vi "BRig_RT__Case_Exp__State_initTrial__LC_Cue__v4.vi"(6 "input_arrTrig":bool[](array[boolean]), 8 "input_dataTrial":u16[][](array[numeric]), 9 "input_dataExp":u16[](array[numeric]), 10 "input_dataLC":u16[](array[numeric]), 11 "input_dataCurrent":u16[](array[numeric])) -> (0 "output_dataTrial":u16[][](array[numeric]), 3 "output_dataCurrent":u16[](array[numeric]), 4 "output_arrTrig":bool[](array[boolean]))   [LabVIEW 2014]
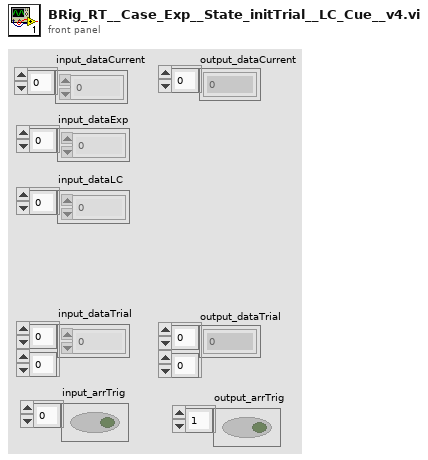
[diagram p1: front panel]
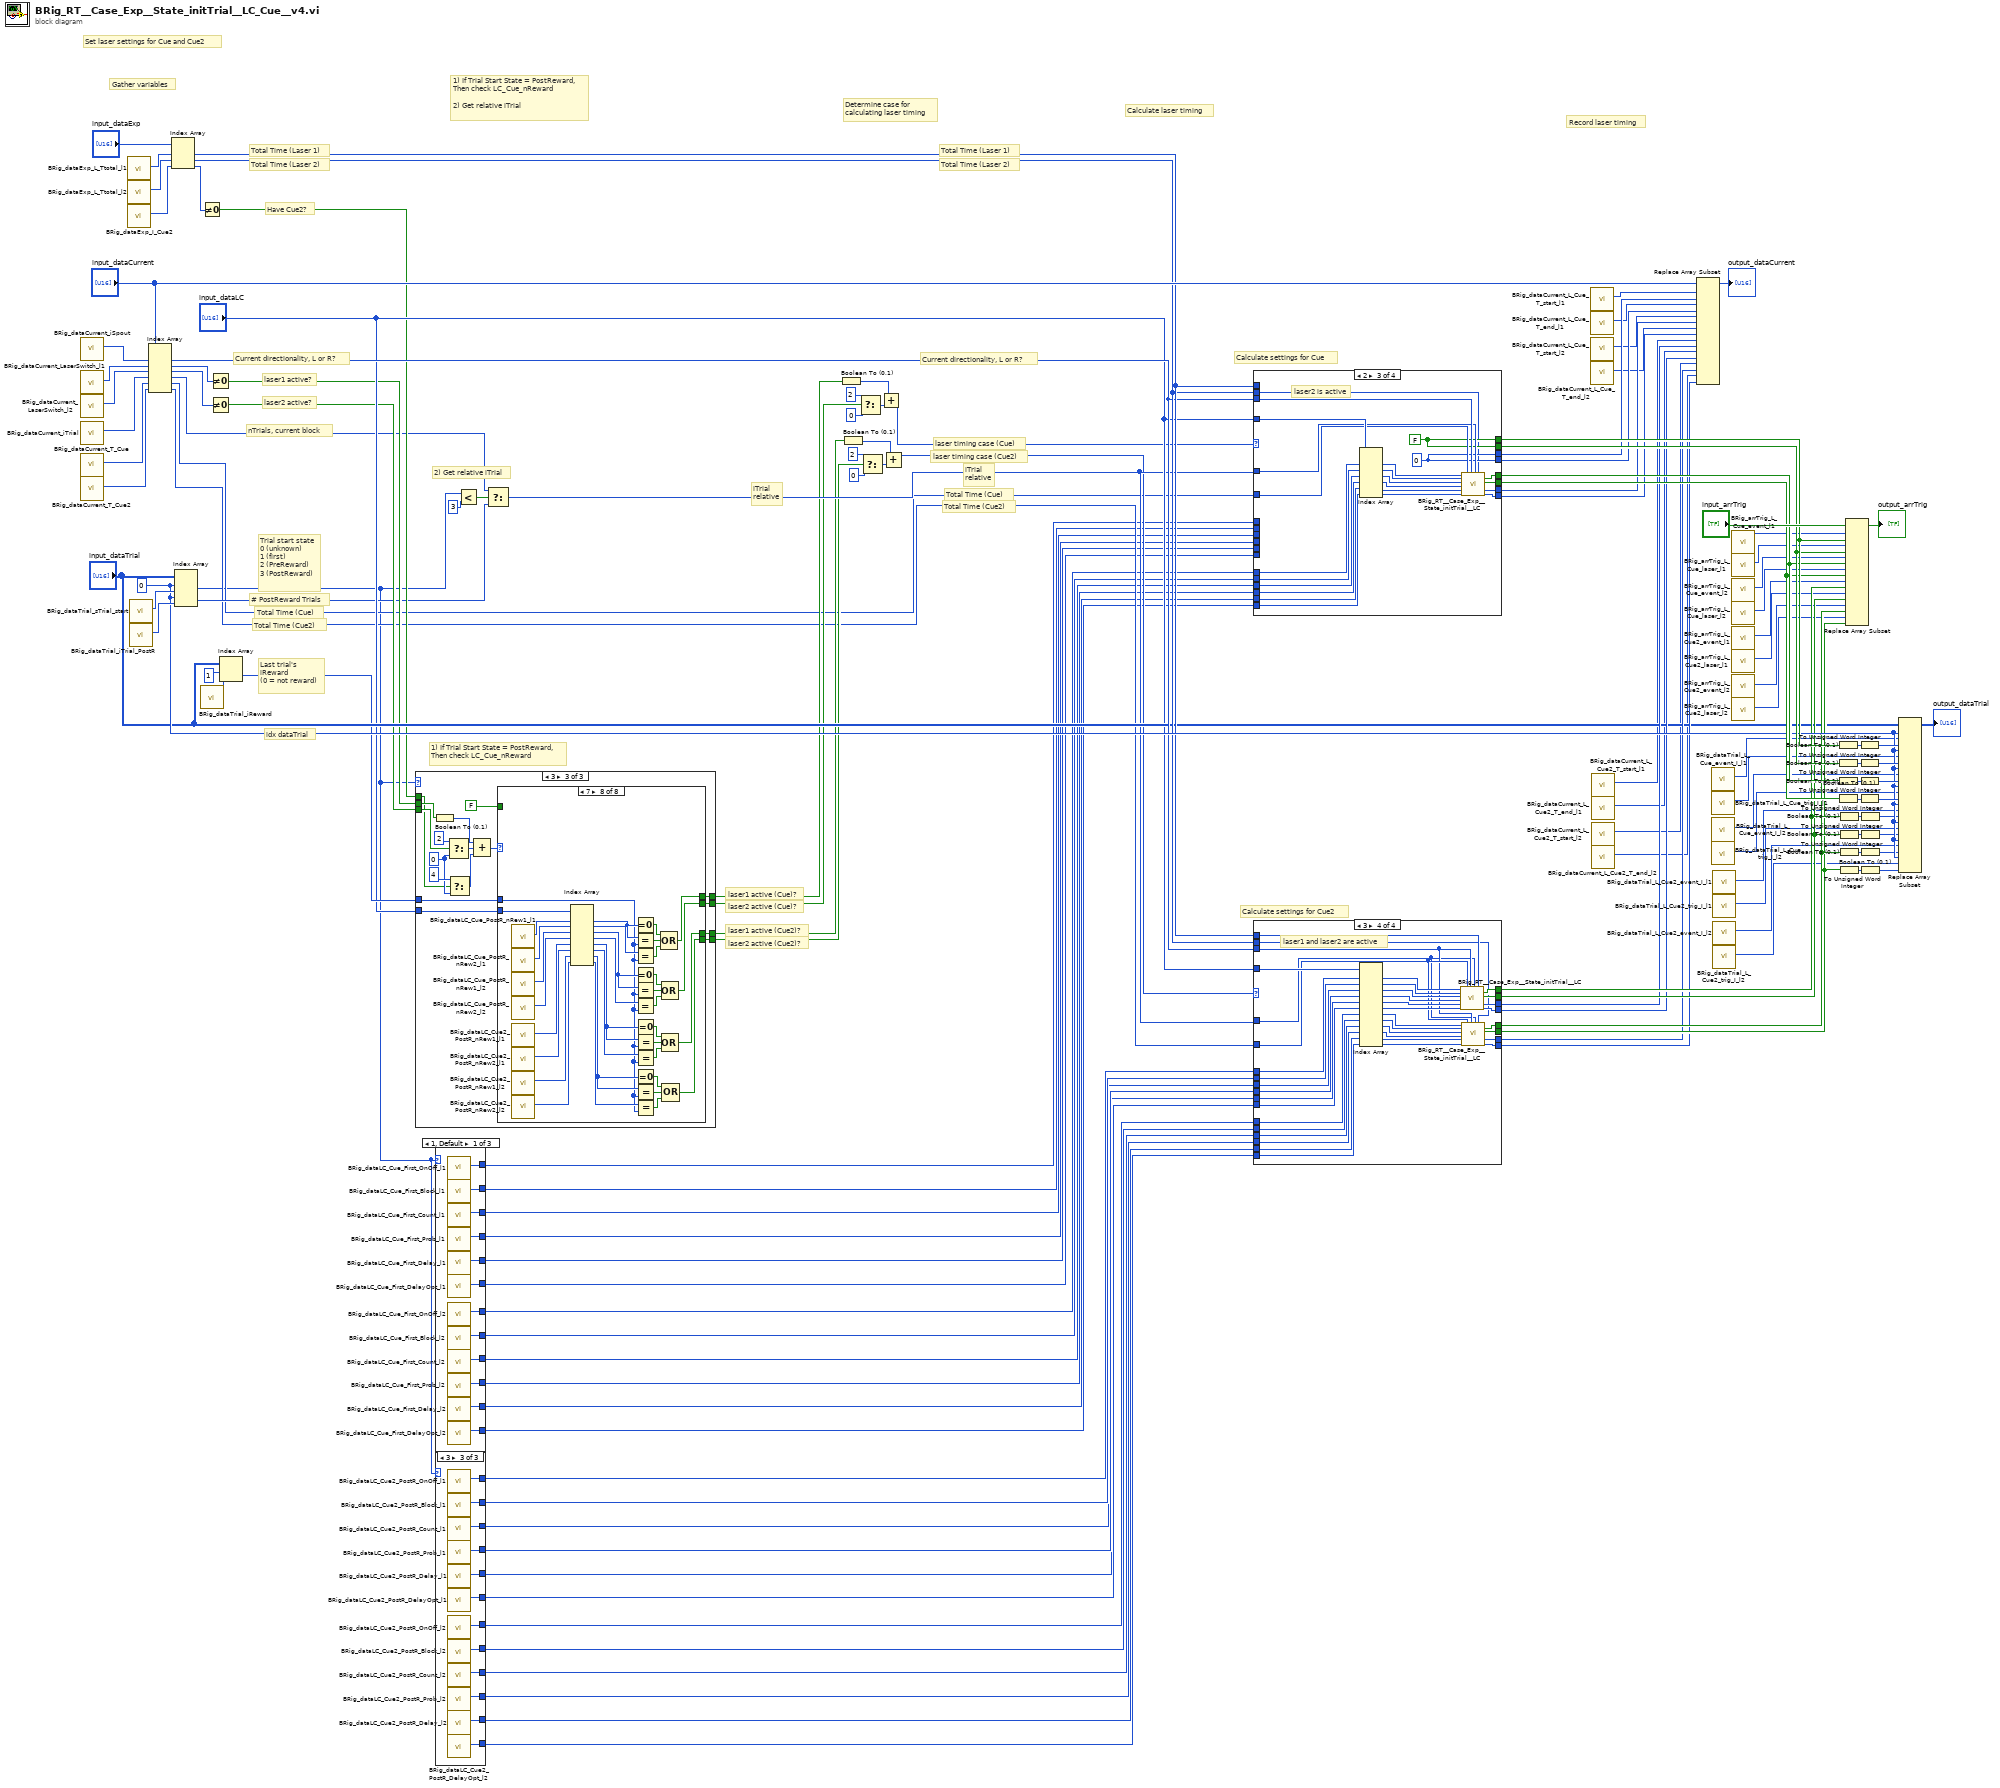
[diagram p0: block diagram]
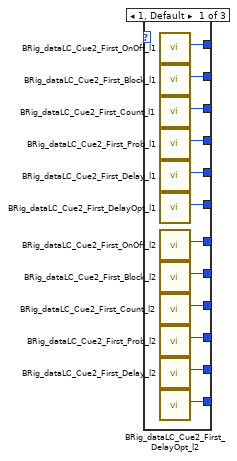
[diagram p2: hidden frame]
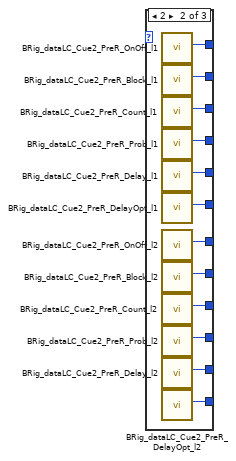
[diagram p3: hidden frame]
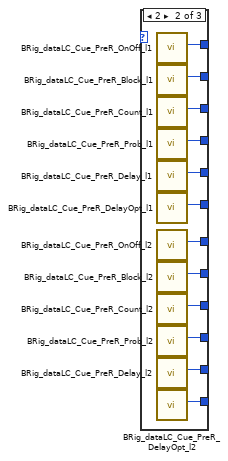
[diagram p4: hidden frame]
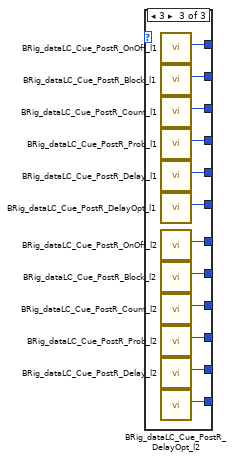
[diagram p5: hidden frame]
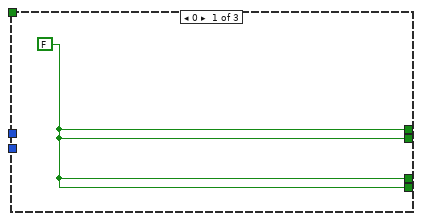
[diagram p6: hidden frame]
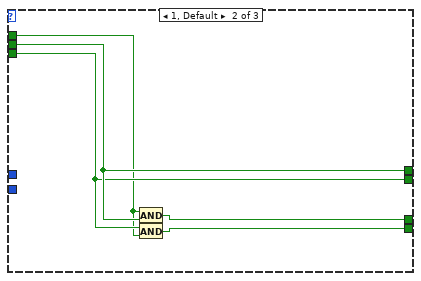
[diagram p7: hidden frame]
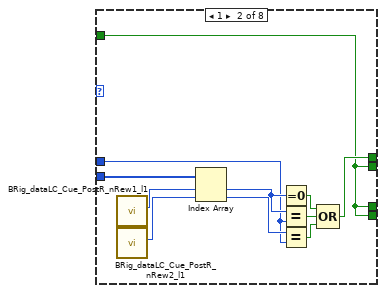
[diagram p9: hidden frame]
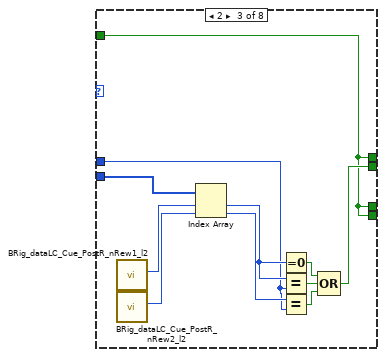
[diagram p10: hidden frame]
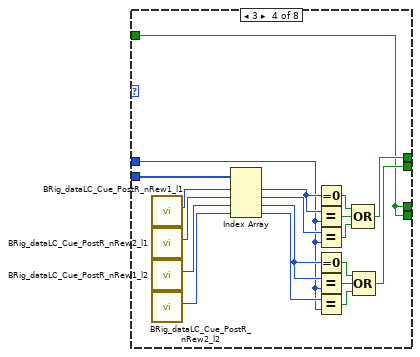
[diagram p11: hidden frame]
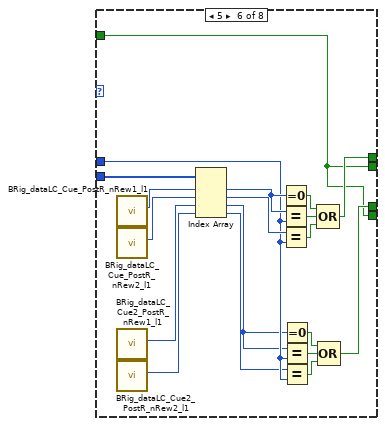
[diagram p13: hidden frame]
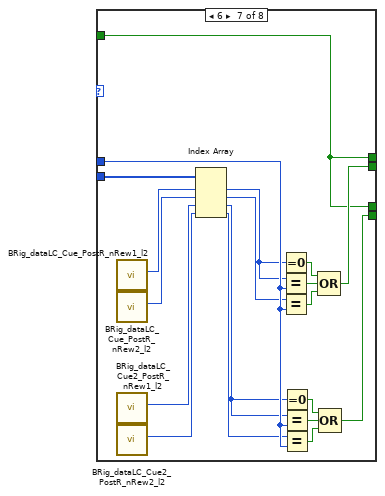
[diagram p14: hidden frame]
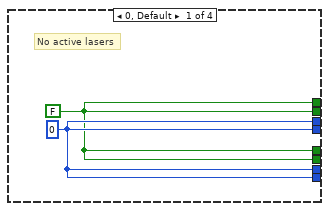
[diagram p15: hidden frame]
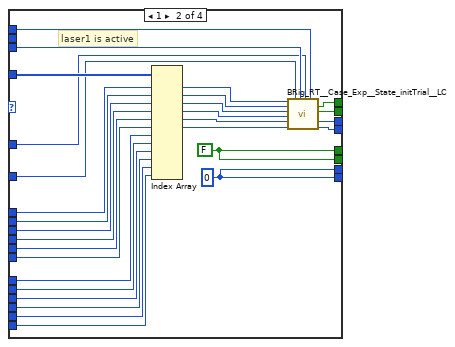
[diagram p16: hidden frame]
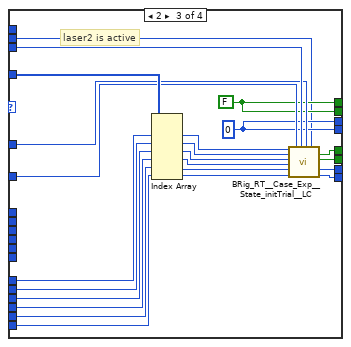
[diagram p17: hidden frame]
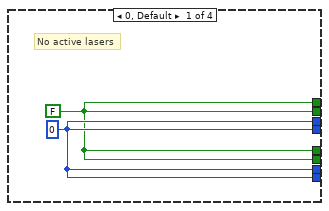
[diagram p18: hidden frame]
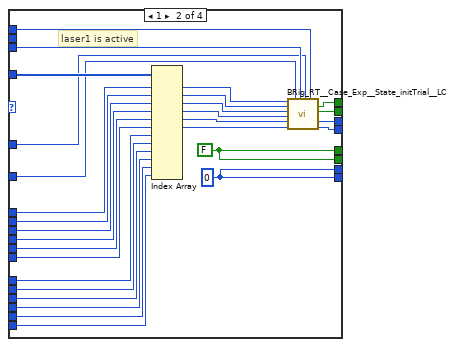
[diagram p19: hidden frame]
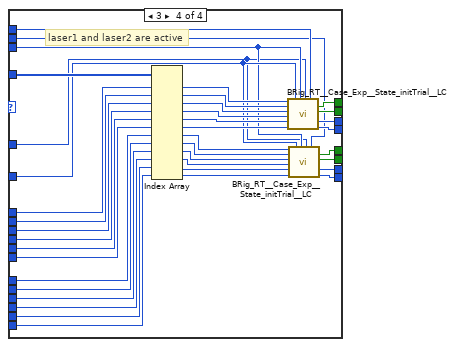
[diagram p20: hidden frame]
diagram:
  w94 = 0
  # "Record laser timing"
  # "Calculate laser timing"
  # "Total Time (Cue2)"
  # "Total Time (Cue)"
  # "iTrial\nrelative"
  # "Total Time (Laser 2)"
  # "Total Time (Laser 1)"
  # "Current directionality, L or R?"
  # "laser timing case (Cue2)"
  # "Determine case for\ncalculating laser timing"
  # "2) Get relative iTrial"
  # "1) If Trial Start State = PostReward,\nThen check LC_Cue_nReward"
  # "laser2 active (Cue2)?"
  # "laser1 active (Cue2)?"
  # "laser2 active (Cue)?"
  # "laser1 active (Cue)?"
  # "1) If Trial Start State = PostReward,\nThen check LC_Cue_nReward\n\n2) Get relative iTrial"
  # "Gather variables"
  # "Last trial's\niReward\n(0 = not reward)"
  # "nTrials, current block"
  # "idx dataTrial"
  # "Total Time (Cue2)"
  # "Total Time (Cue)"
  # "# PostReward Trials"
  # "Current directionality, L or R?"
  # "Have Cue2?"
  # "Total Time (Laser 2)"
  # "Total Time (Laser 1)"
  # "Calculate settings for Cue2"
  # "Calculate settings for Cue"
  # "Set laser settings for Cue and Cue2"
  # "iTrial\nrelative"
  # "laser timing case (Cue)"
  # "Trial start state\n0 (unknown)\n1 (first)\n2 (PreReward)\n3 (PostReward)"
  # "laser2 active?"
  # "laser1 active?"
  n1 = call "BRig_dataCurrent_iSpout.vi"() -> ("output_iSpout"=w125:i32)  [unwired: 11 in]
  n2 = call "BRig_dataCurrent_LaserSwitch_l1.vi"() -> ("output_LaserSwitch_l1"=w134:i32)  [unwired: 11 in]
  n3 = call "BRig_dataCurrent_LaserSwitch_l2.vi"() -> ("output_LaserSwitch_l2"=w133:i32)  [unwired: 11 in]
  n4 = call "BRig_dataCurrent_iTrial.vi"() -> ("output_iTrial"=w99:i32)  [unwired: 11 in]
  n5 = call "BRig_dataCurrent_T_Cue.vi"() -> ("output_T_Cue"=w53:i32)  [unwired: 11 in]
  n6 = call "BRig_dataCurrent_T_Cue2.vi"() -> ("output_T_Cue2"=w52:i32)  [unwired: 11 in]
  n7 = call "BRig_dataExp_L_Ttotal_l1.vi"() -> ("output_L_Ttotal_l1"=w102:i32)  [unwired: 11 in]
  n8 = call "BRig_dataExp_L_Ttotal_l2.vi"() -> ("output_L_Ttotal_l2"=w103:i32)  [unwired: 11 in]
  n9 = call "BRig_dataExp_I_Cue2.vi"() -> ("output_I_Cue2"=w78:i32)  [unwired: 11 in]
  n10 = call "BRig_dataTrial_sTrial_start.vi"() -> ("output_sTrial_start"=w130:i32)  [unwired: 11 in]
  n11 = call "BRig_dataTrial_iTrial_PostR.vi"() -> ("output_iTrial_PostR"=w100:i32)  [unwired: 11 in]
  n12 = Index Array(array="input_dataCurrent", index #1=w125, index #2=w134, index #3=w133, index #4=w99, index #5=w53, index #6=w52) -> (element #1=w87:u16, element #2=w132:u16, element #3=w131:u16, element #4=w66:u16, element #5=w51:u16, element #6=w50:u16)
  n13 = Index Array(array="input_dataExp", index #1=w102, index #2=w103, index #3=w78) -> (element #1=w89:u16, element #2=w88:u16, element #3=w77:u16)
  n14 = Index Array(array="input_dataTrial", index (row) #1=w94, index (col) #1=w130, index (row) #2=w94, index (col) #2=w100) -> (element #1=w25:u16, element #2=w65:u16)
  n15 = Not Equal To 0?(x=w77) -> (x != 0?=w69:bool)
  n16 = call "BRig_dataTrial_iReward.vi"() -> ("output_iReward"=w75:i32)  [unwired: 11 in]
  n17 = Not Equal To 0?(x=w132) -> (x != 0?=w70:bool)
  n18 = Not Equal To 0?(x=w131) -> (x != 0?=w71:bool)
  n19 = Index Array(array="input_dataTrial", index (row)=1 ("disabled index (row)"), index (col)=w75) -> (element=w73:u16)
  n20 = case shown="3" w25 {
    tunnel: w73 -> [_ _ w149]
    tunnel: "input_dataLC" -> [_ _ w150]
    tunnel: w71 -> [_ w139 w142]
    tunnel: w70 -> [_ w140 w143]
    tunnel: w69 -> [_ w138 w141]
    tunnel: [w135 w140 w148] -> w63
    tunnel: [w135 w139 w147] -> w62
    tunnel: [w135 w137 w146] -> w57
    tunnel: [w135 w136 w145] -> w56
    frame 0 {
      w135 = FALSE
    }
    frame 1, Default {
      n21 = And(x=w138, y=w140) -> (x .and. y?=w137:bool)
      n22 = And(x=w139, y=w138) -> (x .and. y?=w136:bool)
    }
    frame 3 {
      w155 = i16 0 ("f")
      n23 = Boolean To (0,1)(Boolean=w143) -> (0, 1=w153:i16)
      n24 = Select(t=i16 2, s=w142, f=w155) -> (s? t:f=w154:i16)
      n25 = Select(t=i16 4, s=w141, f=w155) -> (s? t:f=w152:i16)
      n26 = Compound Arithmetic op=ADD(w153, w154, w152) -> (w151:i16)
      n27 = case shown="7" w151 {
        tunnel: w150 -> [_ w164 w175 w189 _ w214 w235 w262]
        tunnel: w149 -> [_ w163 w174 w188 _ w210 w231 w251]
        tunnel: [w158 w162 w172 w187 w200 w209 w228 w250] -> w148
        tunnel: [w158 w161 w173 w186 w200 w207 w230 w249] -> w147
        tunnel: [w158 w161 w172 w185 w200 w208 w228 w248] -> w146
        tunnel: [w158 w161 w172 w185 w200 w207 w229 w247] -> w145
        tunnel: FALSE -> [w158 w161 w172 w185 w200 w207 w228 _]
        frame 0, Default {
        }
        frame 1 {
          n28 = call "BRig_dataLC_Cue_PostR_nRew1_l1.vi"() -> ("output_Cue_PostR_nRew1_l1"=w159:i32)  [unwired: 11 in]
          n29 = call "BRig_dataLC_Cue_PostR_nRew2_l1.vi"() -> ("output_Cue_PostR_nRew2_l1"=w160:i32)  [unwired: 11 in]
          n30 = Index Array(array=w164, index #1=w159, index #2=w160) -> (element #1=w166:u16, element #2=w165:u16)
          n31 = Equal To 0?(x=w166) -> (x = 0?=w167:bool)
          n32 = Equal?(x=w166, y=w163) -> (x = y?=w168:bool)
          n33 = Equal?(x=w165, y=w163) -> (x = y?=w169:bool)
          n34 = Compound Arithmetic op=OR(w167, w168, w169) -> (w162:bool)
        }
        frame 2 {
          n35 = call "BRig_dataLC_Cue_PostR_nRew1_l2.vi"() -> ("output_Cue_PostR_nRew1_l2"=w170:i32)  [unwired: 11 in]
          n36 = call "BRig_dataLC_Cue_PostR_nRew2_l2.vi"() -> ("output_Cue_PostR_nRew2_l2"=w171:i32)  [unwired: 11 in]
          n37 = Index Array(array=w175, index #1=w170, index #2=w171) -> (element #1=w176:u16, element #2=w177:u16)
          n38 = Equal To 0?(x=w176) -> (x = 0?=w179:bool)
          n39 = Equal?(x=w176, y=w174) -> (x = y?=w178:bool)
          n40 = Equal?(x=w177, y=w174) -> (x = y?=w180:bool)
          n41 = Compound Arithmetic op=OR(w179, w178, w180) -> (w173:bool)
        }
        frame 3 {
          n42 = call "BRig_dataLC_Cue_PostR_nRew1_l1.vi"() -> ("output_Cue_PostR_nRew1_l1"=w181:i32)  [unwired: 11 in]
          n43 = call "BRig_dataLC_Cue_PostR_nRew2_l1.vi"() -> ("output_Cue_PostR_nRew2_l1"=w182:i32)  [unwired: 11 in]
          n44 = call "BRig_dataLC_Cue_PostR_nRew1_l2.vi"() -> ("output_Cue_PostR_nRew1_l2"=w183:i32)  [unwired: 11 in]
          n45 = call "BRig_dataLC_Cue_PostR_nRew2_l2.vi"() -> ("output_Cue_PostR_nRew2_l2"=w184:i32)  [unwired: 11 in]
          n46 = Index Array(array=w189, index #1=w181, index #2=w182, index #3=w183, index #4=w184) -> (element #1=w193:u16, element #2=w192:u16, element #3=w190:u16, element #4=w191:u16)
          n47 = Equal To 0?(x=w193) -> (x = 0?=w194:bool)
          n48 = Equal?(x=w193, y=w188) -> (x = y?=w195:bool)
          n49 = Equal?(x=w192, y=w188) -> (x = y?=w196:bool)
          n50 = Equal To 0?(x=w190) -> (x = 0?=w198:bool)
          n51 = Equal?(x=w190, y=w188) -> (x = y?=w197:bool)
          n52 = Equal?(x=w191, y=w188) -> (x = y?=w199:bool)
          n53 = Compound Arithmetic op=OR(w194, w195, w196) -> (w187:bool)
          n54 = Compound Arithmetic op=OR(w198, w197, w199) -> (w186:bool)
        }
        frame 4 {
        }
        frame 5 {
          n55 = call "BRig_dataLC_Cue_PostR_nRew1_l1.vi"() -> ("output_Cue_PostR_nRew1_l1"=w203:i32)  [unwired: 11 in]
          n56 = call "BRig_dataLC_Cue_PostR_nRew2_l1.vi"() -> ("output_Cue_PostR_nRew2_l1"=w204:i32)  [unwired: 11 in]
          n57 = call "BRig_dataLC_Cue2_PostR_nRew1_l1.vi"() -> ("output_Cue2_PostR_nRew1_l1"=w201:i32)  [unwired: 11 in]
          n58 = call "BRig_dataLC_Cue2_PostR_nRew2_l1.vi"() -> ("output_Cue2_PostR_nRew2_l1"=w202:i32)  [unwired: 11 in]
          n59 = Index Array(array=w214, index #1=w203, index #2=w204, index #3=w201, index #4=w202) -> (element #1=w216:u16, element #2=w215:u16, element #3=w206:u16, element #4=w205:u16)
          n60 = Equal To 0?(x=w216) -> (x = 0?=w217:bool)
          n61 = Equal?(x=w216, y=w210) -> (x = y?=w218:bool)
          n62 = Equal?(x=w215, y=w210) -> (x = y?=w219:bool)
          n63 = Equal To 0?(x=w206) -> (x = 0?=w213:bool)
          n64 = Equal?(x=w206, y=w210) -> (x = y?=w212:bool)
          n65 = Equal?(x=w205, y=w210) -> (x = y?=w211:bool)
          n66 = Compound Arithmetic op=OR(w217, w218, w219) -> (w209:bool)
          n67 = Compound Arithmetic op=OR(w213, w212, w211) -> (w208:bool)
        }
        frame 6 {
          n68 = call "BRig_dataLC_Cue_PostR_nRew1_l2.vi"() -> ("output_Cue_PostR_nRew1_l2"=w223:i32)  [unwired: 11 in]
          n69 = call "BRig_dataLC_Cue_PostR_nRew2_l2.vi"() -> ("output_Cue_PostR_nRew2_l2"=w222:i32)  [unwired: 11 in]
          n70 = call "BRig_dataLC_Cue2_PostR_nRew1_l2.vi"() -> ("output_Cue2_PostR_nRew1_l2"=w221:i32)  [unwired: 11 in]
          n71 = call "BRig_dataLC_Cue2_PostR_nRew2_l2.vi"() -> ("output_Cue2_PostR_nRew2_l2"=w220:i32)  [unwired: 11 in]
          n72 = Index Array(array=w235, index #1=w223, index #2=w222, index #3=w221, index #4=w220) -> (element #1=w227:u16, element #2=w226:u16, element #3=w225:u16, element #4=w224:u16)
          n73 = Equal To 0?(x=w227) -> (x = 0?=w237:bool)
          n74 = Equal?(x=w227, y=w231) -> (x = y?=w236:bool)
          n75 = Equal?(x=w226, y=w231) -> (x = y?=w238:bool)
          n76 = Equal To 0?(x=w225) -> (x = 0?=w233:bool)
          n77 = Equal?(x=w225, y=w231) -> (x = y?=w234:bool)
          n78 = Equal?(x=w224, y=w231) -> (x = y?=w232:bool)
          n79 = Compound Arithmetic op=OR(w237, w236, w238) -> (w230:bool)
          n80 = Compound Arithmetic op=OR(w233, w234, w232) -> (w229:bool)
        }
        frame 7 {
          n81 = call "BRig_dataLC_Cue_PostR_nRew1_l1.vi"() -> ("output_Cue_PostR_nRew1_l1"=w243:i32)  [unwired: 11 in]
          n82 = call "BRig_dataLC_Cue_PostR_nRew2_l1.vi"() -> ("output_Cue_PostR_nRew2_l1"=w244:i32)  [unwired: 11 in]
          n83 = call "BRig_dataLC_Cue_PostR_nRew1_l2.vi"() -> ("output_Cue_PostR_nRew1_l2"=w245:i32)  [unwired: 11 in]
          n84 = call "BRig_dataLC_Cue_PostR_nRew2_l2.vi"() -> ("output_Cue_PostR_nRew2_l2"=w246:i32)  [unwired: 11 in]
          n85 = call "BRig_dataLC_Cue2_PostR_nRew1_l1.vi"() -> ("output_Cue2_PostR_nRew1_l1"=w242:i32)  [unwired: 11 in]
          n86 = call "BRig_dataLC_Cue2_PostR_nRew2_l1.vi"() -> ("output_Cue2_PostR_nRew2_l1"=w241:i32)  [unwired: 11 in]
          n87 = call "BRig_dataLC_Cue2_PostR_nRew1_l2.vi"() -> ("output_Cue2_PostR_nRew1_l2"=w240:i32)  [unwired: 11 in]
          n88 = call "BRig_dataLC_Cue2_PostR_nRew2_l2.vi"() -> ("output_Cue2_PostR_nRew2_l2"=w239:i32)  [unwired: 11 in]
          n89 = Index Array(array=w262, index #1=w243, index #2=w244, index #3=w245, index #4=w246, index #5=w242, index #6=w241, index #7=w240, index #8=w239) -> (element #1=w266:u16, element #2=w265:u16, element #3=w263:u16, element #4=w264:u16, element #5=w255:u16, element #6=w254:u16, element #7=w252:u16, element #8=w253:u16)
          n90 = Equal To 0?(x=w266) -> (x = 0?=w267:bool)
          n91 = Equal?(x=w266, y=w251) -> (x = y?=w268:bool)
          n92 = Equal?(x=w265, y=w251) -> (x = y?=w269:bool)
          n93 = Equal To 0?(x=w263) -> (x = 0?=w271:bool)
          n94 = Equal?(x=w263, y=w251) -> (x = y?=w270:bool)
          n95 = Equal?(x=w264, y=w251) -> (x = y?=w272:bool)
          n96 = Equal To 0?(x=w255) -> (x = 0?=w261:bool)
          n97 = Equal?(x=w255, y=w251) -> (x = y?=w260:bool)
          n98 = Equal?(x=w254, y=w251) -> (x = y?=w259:bool)
          n99 = Equal To 0?(x=w252) -> (x = 0?=w257:bool)
          n100 = Equal?(x=w252, y=w251) -> (x = y?=w258:bool)
          n101 = Equal?(x=w253, y=w251) -> (x = y?=w256:bool)
          n102 = Compound Arithmetic op=OR(w267, w268, w269) -> (w250:bool)
          n103 = Compound Arithmetic op=OR(w271, w270, w272) -> (w249:bool)
          n104 = Compound Arithmetic op=OR(w261, w260, w259) -> (w248:bool)
          n105 = Compound Arithmetic op=OR(w257, w258, w256) -> (w247:bool)
        }
      }
    }
  }
  n106 = case shown="1, Default" w25 {
    tunnel: [w273 w296 w307] -> w38
    tunnel: [w274 w285 w306] -> w39
    tunnel: [w275 w286 w305] -> w40
    tunnel: [w276 w287 w304] -> w41
    tunnel: [w277 w288 w303] -> w42
    tunnel: [w278 w289 w302] -> w43
    tunnel: [w279 w295 w301] -> w44
    tunnel: [w280 w290 w300] -> w45
    tunnel: [w281 w291 w299] -> w46
    tunnel: [w282 w292 w298] -> w47
    tunnel: [w283 w293 w297] -> w48
    tunnel: [w284 w294 w308] -> w49
    frame 1, Default {
      n107 = call "BRig_dataLC_Cue_First_OnOff_l1.vi"() -> ("output_Cue_First_OnOff"=w273:i32)  [unwired: 11 in]
      n108 = call "BRig_dataLC_Cue_First_Block_l1.vi"() -> ("output_Cue_First_Block"=w274:i32)  [unwired: 11 in]
      n109 = call "BRig_dataLC_Cue_First_Count_l1.vi"() -> ("output_Cue_First_Count"=w275:i32)  [unwired: 11 in]
      n110 = call "BRig_dataLC_Cue_First_Prob_l1.vi"() -> ("output_Cue_First_Prob"=w276:i32)  [unwired: 11 in]
      n111 = call "BRig_dataLC_Cue_First_Delay_l1.vi"() -> ("output_Cue_First_Delay"=w277:i32)  [unwired: 11 in]
      n112 = call "BRig_dataLC_Cue_First_DelayOpt_l1.vi"() -> ("output_Cue_First_DelayOpt"=w278:i32)  [unwired: 11 in]
      n113 = call "BRig_dataLC_Cue_First_OnOff_l2.vi"() -> ("output_Cue_First_OnOff_l2"=w279:i32)  [unwired: 11 in]
      n114 = call "BRig_dataLC_Cue_First_Block_l2.vi"() -> ("output_Cue_First_Block_l2"=w280:i32)  [unwired: 11 in]
      n115 = call "BRig_dataLC_Cue_First_Count_l2.vi"() -> ("output_Cue_First_Count_l2"=w281:i32)  [unwired: 11 in]
      n116 = call "BRig_dataLC_Cue_First_Prob_l2.vi"() -> ("output_Cue_First_Prob_l2"=w282:i32)  [unwired: 11 in]
      n117 = call "BRig_dataLC_Cue_First_Delay_l2.vi"() -> ("output_Cue_First_Delay_l2"=w283:i32)  [unwired: 11 in]
      n118 = call "BRig_dataLC_Cue_First_DelayOpt_l2.vi"() -> ("output_Cue_First_DelayOpt_l2"=w284:i32)  [unwired: 11 in]
    }
    frame 2 {
      n119 = call "BRig_dataLC_Cue_PreR_OnOff_l1.vi"() -> ("output_Cue_PreR_OnOff"=w296:i32)  [unwired: 11 in]
      n120 = call "BRig_dataLC_Cue_PreR_Block_l1.vi"() -> ("output_Cue_PreR_Block"=w285:i32)  [unwired: 11 in]
      n121 = call "BRig_dataLC_Cue_PreR_Count_l1.vi"() -> ("output_Cue_PreR_Count"=w286:i32)  [unwired: 11 in]
      n122 = call "BRig_dataLC_Cue_PreR_Prob_l1.vi"() -> ("output_Cue_PreR_Prob"=w287:i32)  [unwired: 11 in]
      n123 = call "BRig_dataLC_Cue_PreR_Delay_l1.vi"() -> ("output_Cue_PreR_Delay"=w288:i32)  [unwired: 11 in]
      n124 = call "BRig_dataLC_Cue_PreR_DelayOpt_l1.vi"() -> ("output_Cue_PreR_DelayOpt"=w289:i32)  [unwired: 11 in]
      n125 = call "BRig_dataLC_Cue_PreR_OnOff_l2.vi"() -> ("output_Cue_PreR_OnOff_l2"=w295:i32)  [unwired: 11 in]
      n126 = call "BRig_dataLC_Cue_PreR_Block_l2.vi"() -> ("output_Cue_PreR_Block_l2"=w290:i32)  [unwired: 11 in]
      n127 = call "BRig_dataLC_Cue_PreR_Count_l2.vi"() -> ("output_Cue_PreR_Count_l2"=w291:i32)  [unwired: 11 in]
      n128 = call "BRig_dataLC_Cue_PreR_Prob_l2.vi"() -> ("output_Cue_PreR_Prob_l2"=w292:i32)  [unwired: 11 in]
      n129 = call "BRig_dataLC_Cue_PreR_Delay_l2.vi"() -> ("output_Cue_PreR_Delay_l2"=w293:i32)  [unwired: 11 in]
      n130 = call "BRig_dataLC_Cue_PreR_DelayOpt_l2.vi"() -> ("output_Cue_PreR_DelayOpt_l2"=w294:i32)  [unwired: 11 in]
    }
    frame 3 {
      n131 = call "BRig_dataLC_Cue_PostR_OnOff_l1.vi"() -> ("output_Cue_PostR_OnOff"=w307:i32)  [unwired: 11 in]
      n132 = call "BRig_dataLC_Cue_PostR_Block_l1.vi"() -> ("output_Cue_PostR_Block"=w306:i32)  [unwired: 11 in]
      n133 = call "BRig_dataLC_Cue_PostR_Count_l1.vi"() -> ("output_Cue_PostR_Count"=w305:i32)  [unwired: 11 in]
      n134 = call "BRig_dataLC_Cue_PostR_Prob_l1.vi"() -> ("output_Cue_PostR_Prob"=w304:i32)  [unwired: 11 in]
      n135 = call "BRig_dataLC_Cue_PostR_Delay_l1.vi"() -> ("output_Cue_PostR_Delay"=w303:i32)  [unwired: 11 in]
      n136 = call "BRig_dataLC_Cue_PostR_DelayOpt_l1.vi"() -> ("output_Cue_PostR_DelayOpt"=w302:i32)  [unwired: 11 in]
      n137 = call "BRig_dataLC_Cue_PostR_OnOff_l2.vi"() -> ("output_Cue_PostR_OnOff_l2"=w301:i32)  [unwired: 11 in]
      n138 = call "BRig_dataLC_Cue_PostR_Block_l2.vi"() -> ("output_Cue_PostR_Block_l2"=w300:i32)  [unwired: 11 in]
      n139 = call "BRig_dataLC_Cue_PostR_Count_l2.vi"() -> ("output_Cue_PostR_Count_l2"=w299:i32)  [unwired: 11 in]
      n140 = call "BRig_dataLC_Cue_PostR_Prob_l2.vi"() -> ("output_Cue_PostR_Prob_l2"=w298:i32)  [unwired: 11 in]
      n141 = call "BRig_dataLC_Cue_PostR_Delay_l2.vi"() -> ("output_Cue_PostR_Delay_l2"=w297:i32)  [unwired: 11 in]
      n142 = call "BRig_dataLC_Cue_PostR_DelayOpt_l2.vi"() -> ("output_Cue_PostR_DelayOpt_l2"=w308:i32)  [unwired: 11 in]
    }
  }
  n143 = case shown="3" w25 {
    tunnel: [w320 w332 w344] -> w37
    tunnel: [w319 w331 w343] -> w36
    tunnel: [w318 w330 w342] -> w35
    tunnel: [w317 w329 w341] -> w34
    tunnel: [w316 w328 w340] -> w33
    tunnel: [w315 w327 w339] -> w32
    tunnel: [w314 w326 w338] -> w31
    tunnel: [w313 w325 w337] -> w30
    tunnel: [w312 w324 w336] -> w29
    tunnel: [w311 w323 w335] -> w28
    tunnel: [w310 w322 w334] -> w27
    tunnel: [w309 w321 w333] -> w26
    frame 1, Default {
      n144 = call "BRig_dataLC_Cue2_First_OnOff_l1.vi"() -> ("output_Cue2_First_OnOff"=w320:i32)  [unwired: 11 in]
      n145 = call "BRig_dataLC_Cue2_First_Block_l1.vi"() -> ("output_Cue2_First_Block"=w319:i32)  [unwired: 11 in]
      n146 = call "BRig_dataLC_Cue2_First_Count_l1.vi"() -> ("output_Cue2_First_Count"=w318:i32)  [unwired: 11 in]
      n147 = call "BRig_dataLC_Cue2_First_Prob_l1.vi"() -> ("output_Cue2_First_Prob"=w317:i32)  [unwired: 11 in]
      n148 = call "BRig_dataLC_Cue2_First_Delay_l1.vi"() -> ("output_Cue2_First_Delay"=w316:i32)  [unwired: 11 in]
      n149 = call "BRig_dataLC_Cue2_First_DelayOpt_l1.vi"() -> ("output_Cue2_First_DelayOpt"=w315:i32)  [unwired: 11 in]
      n150 = call "BRig_dataLC_Cue2_First_OnOff_l2.vi"() -> ("output_Cue2_First_OnOff_l2"=w314:i32)  [unwired: 11 in]
      n151 = call "BRig_dataLC_Cue2_First_Block_l2.vi"() -> ("output_Cue2_First_Block_l2"=w313:i32)  [unwired: 11 in]
      n152 = call "BRig_dataLC_Cue2_First_Count_l2.vi"() -> ("output_Cue2_First_Count_l2"=w312:i32)  [unwired: 11 in]
      n153 = call "BRig_dataLC_Cue2_First_Prob_l2.vi"() -> ("output_Cue2_First_Prob_l2"=w311:i32)  [unwired: 11 in]
      n154 = call "BRig_dataLC_Cue2_First_Delay_l2.vi"() -> ("output_Cue2_First_Delay_l2"=w310:i32)  [unwired: 11 in]
      n155 = call "BRig_dataLC_Cue2_First_DelayOpt_l2.vi"() -> ("output_Cue2_First_DelayOpt_l2"=w309:i32)  [unwired: 11 in]
    }
    frame 2 {
      n156 = call "BRig_dataLC_Cue2_PreR_OnOff_l1.vi"() -> ("output_Cue2_PreR_OnOff"=w332:i32)  [unwired: 11 in]
      n157 = call "BRig_dataLC_Cue2_PreR_Block_l1.vi"() -> ("output_Cue2_PreR_Block"=w331:i32)  [unwired: 11 in]
      n158 = call "BRig_dataLC_Cue2_PreR_Count_l1.vi"() -> ("output_Cue2_PreR_Count"=w330:i32)  [unwired: 11 in]
      n159 = call "BRig_dataLC_Cue2_PreR_Prob_l1.vi"() -> ("output_Cue2_PreR_Prob"=w329:i32)  [unwired: 11 in]
      n160 = call "BRig_dataLC_Cue2_PreR_Delay_l1.vi"() -> ("output_Cue2_PreR_Delay"=w328:i32)  [unwired: 11 in]
      n161 = call "BRig_dataLC_Cue2_PreR_DelayOpt_l1.vi"() -> ("output_Cue2_PreR_DelayOpt"=w327:i32)  [unwired: 11 in]
      n162 = call "BRig_dataLC_Cue2_PreR_OnOff_l2.vi"() -> ("output_Cue2_PreR_OnOff_l2"=w326:i32)  [unwired: 11 in]
      n163 = call "BRig_dataLC_Cue2_PreR_Block_l2.vi"() -> ("output_Cue2_PreR_Block_l2"=w325:i32)  [unwired: 11 in]
      n164 = call "BRig_dataLC_Cue2_PreR_Count_l2.vi"() -> ("output_Cue2_PreR_Count_l2"=w324:i32)  [unwired: 11 in]
      n165 = call "BRig_dataLC_Cue2_PreR_Prob_l2.vi"() -> ("output_Cue2_PreR_Prob_l2"=w323:i32)  [unwired: 11 in]
      n166 = call "BRig_dataLC_Cue2_PreR_Delay_l2.vi"() -> ("output_Cue2_PreR_Delay_l2"=w322:i32)  [unwired: 11 in]
      n167 = call "BRig_dataLC_Cue2_PreR_DelayOpt_l2.vi"() -> ("output_Cue2_PreR_DelayOpt_l2"=w321:i32)  [unwired: 11 in]
    }
    frame 3 {
      n168 = call "BRig_dataLC_Cue2_PostR_OnOff_l1.vi"() -> ("output_Cue2_PostR_OnOff"=w344:i32)  [unwired: 11 in]
      n169 = call "BRig_dataLC_Cue2_PostR_Block_l1.vi"() -> ("output_Cue2_PostR_Block"=w343:i32)  [unwired: 11 in]
      n170 = call "BRig_dataLC_Cue2_PostR_Count_l1.vi"() -> ("output_Cue2_PostR_Count"=w342:i32)  [unwired: 11 in]
      n171 = call "BRig_dataLC_Cue2_PostR_Prob_l1.vi"() -> ("output_Cue2_PostR_Prob"=w341:i32)  [unwired: 11 in]
      n172 = call "BRig_dataLC_Cue2_PostR_Delay_l1.vi"() -> ("output_Cue2_PostR_Delay"=w340:i32)  [unwired: 11 in]
      n173 = call "BRig_dataLC_Cue2_PostR_DelayOpt_l1.vi"() -> ("output_Cue2_PostR_DelayOpt"=w339:i32)  [unwired: 11 in]
      n174 = call "BRig_dataLC_Cue2_PostR_OnOff_l2.vi"() -> ("output_Cue2_PostR_OnOff_l2"=w338:i32)  [unwired: 11 in]
      n175 = call "BRig_dataLC_Cue2_PostR_Block_l2.vi"() -> ("output_Cue2_PostR_Block_l2"=w337:i32)  [unwired: 11 in]
      n176 = call "BRig_dataLC_Cue2_PostR_Count_l2.vi"() -> ("output_Cue2_PostR_Count_l2"=w336:i32)  [unwired: 11 in]
      n177 = call "BRig_dataLC_Cue2_PostR_Prob_l2.vi"() -> ("output_Cue2_PostR_Prob_l2"=w335:i32)  [unwired: 11 in]
      n178 = call "BRig_dataLC_Cue2_PostR_Delay_l2.vi"() -> ("output_Cue2_PostR_Delay_l2"=w334:i32)  [unwired: 11 in]
      n179 = call "BRig_dataLC_Cue2_PostR_DelayOpt_l2.vi"() -> ("output_Cue2_PostR_DelayOpt_l2"=w333:i32)  [unwired: 11 in]
    }
  }
  n180 = Less?(x=w25, y=u16 3) -> (x < y?=w67:bool)
  n181 = Select(t=w66, s=w67, f=w65) -> (s? t:f=w64:u16)
  n182 = Boolean To (0,1)(Boolean=w63) -> (0, 1=w127:i16)
  n183 = Boolean To (0,1)(Boolean=w57) -> (0, 1=w60:i16)
  n184 = Select(t=i16 2, s=w62, f=i16 0) -> (s? t:f=w128:i16)
  n185 = Select(t=i16 2, s=w56, f=i16 0) -> (s? t:f=w59:i16)
  n186 = Add(x=w127, y=w128) -> (x+y=w55:i16)
  n187 = Add(x=w60, y=w59) -> (x+y=w54:i16)
  n188 = case shown="2" w55 {
    tunnel: "input_dataLC" -> [_ w375 w398 w436]
    tunnel: w87 -> [_ w367 w390 w422]
    tunnel: w51 -> [_ w368 w391 w423]
    tunnel: w64 -> [_ w366 w389 w421]
    tunnel: [w345 w365 w378 w420] -> w118
    tunnel: [w345 w364 w378 w419] -> w115
    tunnel: [w346 w363 w377 w418] -> w107
    tunnel: [w346 w362 w377 w417] -> w106
    tunnel: [w345 w349 w388 w416] -> w111
    tunnel: [w346 w348 w387 w415] -> w105
    tunnel: [w345 w349 w386 w414] -> w113
    tunnel: [w346 w348 w385 w413] -> w104
    tunnel: w38 -> [_ w361 _ w412]
    tunnel: w39 -> [_ w360 _ w411]
    tunnel: w40 -> [_ w359 _ w410]
    tunnel: w41 -> [_ w358 _ w409]
    tunnel: w42 -> [_ w357 _ w408]
    tunnel: w43 -> [_ w356 _ w407]
    tunnel: w44 -> [_ w355 w384 w406]
    tunnel: w45 -> [_ w354 w383 w405]
    tunnel: w46 -> [_ w353 w382 w404]
    tunnel: w47 -> [_ w352 w381 w403]
    tunnel: w48 -> [_ w351 w380 w402]
    tunnel: w49 -> [_ w350 w379 w401]
    tunnel: w89 -> [_ w347 _ w400]
    tunnel: w88 -> [_ _ w376 w399]
    frame 0, Default {
      w346 = u16 0
      w345 = FALSE
      # "No active lasers"
    }
    frame 1 {
      w348 = u16 0
      w349 = FALSE
      # "laser1 is active"
      n189 = Index Array(array=w375, index #1=w361, index #2=w360, index #3=w359, index #4=w358, index #5=w357, index #6=w356, index #7=w355, index #8=w354, index #9=w353, index #10=w352, index #11=w351, index #12=w350) -> (element #1=w374:u16, element #2=w373:u16, element #3=w372:u16, element #4=w371:u16, element #5=w370:u16, element #6=w369:u16)  [unwired: 6 out]
      n190 = call "BRig_RT__Case_Exp__State_initTrial__LC.vi"("input_L_OnOff"=w374, "input_L_Block"=w373, "input_L_Count"=w372, "input_L_Prob"=w371, "input_L_Tdelay"=w370, "input_L_delayOpt"=w369, "input_T_state"=w368, "input_iSpout"=w367, "input_iTrial_relative"=w366, "input_L_T"=w347) -> ("output_LC_Event"=w365:bool, "output_LC_Laser"=w364:bool, "output_L_Tstart"=w363:u16, "output_L_Tend"=w362:u16)  [unwired: 6 in]
    }
    frame 2 {
      w377 = u16 0
      w378 = FALSE
      # "laser2 is active"
      n191 = Index Array(array=w398, index #1=w384, index #2=w383, index #3=w382, index #4=w381, index #5=w380, index #6=w379) -> (element #1=w392:u16, element #2=w393:u16, element #3=w394:u16, element #4=w395:u16, element #5=w396:u16, element #6=w397:u16)
      n192 = call "BRig_RT__Case_Exp__State_initTrial__LC.vi"("input_L_OnOff"=w392, "input_L_Block"=w393, "input_L_Count"=w394, "input_L_Prob"=w395, "input_L_Tdelay"=w396, "input_L_delayOpt"=w397, "input_T_state"=w391, "input_iSpout"=w390, "input_iTrial_relative"=w389, "input_L_T"=w376) -> ("output_LC_Event"=w386:bool, "output_LC_Laser"=w388:bool, "output_L_Tstart"=w387:u16, "output_L_Tend"=w385:u16)  [unwired: 6 in]
    }
    frame 3 {
      # "laser1 and laser2 are active"
      n193 = Index Array(array=w436, index #1=w412, index #2=w411, index #3=w410, index #4=w409, index #5=w408, index #6=w407, index #7=w406, index #8=w405, index #9=w404, index #10=w403, index #11=w402, index #12=w401) -> (element #1=w435:u16, element #2=w434:u16, element #3=w433:u16, element #4=w432:u16, element #5=w431:u16, element #6=w430:u16, element #7=w424:u16, element #8=w425:u16, element #9=w426:u16, element #10=w427:u16, element #11=w428:u16, element #12=w429:u16)
      n194 = call "BRig_RT__Case_Exp__State_initTrial__LC.vi"("input_L_OnOff"=w435, "input_L_Block"=w434, "input_L_Count"=w433, "input_L_Prob"=w432, "input_L_Tdelay"=w431, "input_L_delayOpt"=w430, "input_T_state"=w423, "input_iSpout"=w422, "input_iTrial_relative"=w421, "input_L_T"=w400) -> ("output_LC_Event"=w420:bool, "output_LC_Laser"=w419:bool, "output_L_Tstart"=w418:u16, "output_L_Tend"=w417:u16)  [unwired: 6 in]
      n195 = call "BRig_RT__Case_Exp__State_initTrial__LC.vi"("input_L_OnOff"=w424, "input_L_Block"=w425, "input_L_Count"=w426, "input_L_Prob"=w427, "input_L_Tdelay"=w428, "input_L_delayOpt"=w429, "input_T_state"=w423, "input_iSpout"=w422, "input_iTrial_relative"=w421, "input_L_T"=w399) -> ("output_LC_Event"=w414:bool, "output_LC_Laser"=w416:bool, "output_L_Tstart"=w415:u16, "output_L_Tend"=w413:u16)  [unwired: 6 in]
    }
  }
  n196 = case shown="3" w54 {
    tunnel: "input_dataLC" -> [_ w467 w490 w528]
    tunnel: w87 -> [_ w459 w482 w514]
    tunnel: w50 -> [_ w460 w483 w515]
    tunnel: w64 -> [_ w458 w481 w513]
    tunnel: [w437 w457 w470 w512] -> w86
    tunnel: [w437 w456 w470 w511] -> w85
    tunnel: [w438 w455 w469 w510] -> w82
    tunnel: [w438 w454 w469 w509] -> w81
    tunnel: [w437 w441 w480 w508] -> w83
    tunnel: [w438 w440 w479 w507] -> w80
    tunnel: [w437 w441 w478 w506] -> w84
    tunnel: [w438 w440 w477 w505] -> w79
    tunnel: w37 -> [_ w453 _ w504]
    tunnel: w36 -> [_ w452 _ w503]
    tunnel: w35 -> [_ w451 _ w502]
    tunnel: w34 -> [_ w450 _ w501]
    tunnel: w33 -> [_ w449 _ w500]
    tunnel: w32 -> [_ w448 _ w499]
    tunnel: w31 -> [_ w447 w476 w498]
    tunnel: w30 -> [_ w446 w475 w497]
    tunnel: w29 -> [_ w445 w474 w496]
    tunnel: w28 -> [_ w444 w473 w495]
    tunnel: w27 -> [_ w443 w472 w494]
    tunnel: w26 -> [_ w442 w471 w493]
    tunnel: w89 -> [_ w439 _ w492]
    tunnel: w88 -> [_ _ w468 w491]
    frame 0, Default {
      w438 = u16 0
      w437 = FALSE
      # "No active lasers"
    }
    frame 1 {
      w440 = u16 0
      w441 = FALSE
      # "laser1 is active"
      n197 = Index Array(array=w467, index #1=w453, index #2=w452, index #3=w451, index #4=w450, index #5=w449, index #6=w448, index #7=w447, index #8=w446, index #9=w445, index #10=w444, index #11=w443, index #12=w442) -> (element #1=w466:u16, element #2=w465:u16, element #3=w464:u16, element #4=w463:u16, element #5=w462:u16, element #6=w461:u16)  [unwired: 6 out]
      n198 = call "BRig_RT__Case_Exp__State_initTrial__LC.vi"("input_L_OnOff"=w466, "input_L_Block"=w465, "input_L_Count"=w464, "input_L_Prob"=w463, "input_L_Tdelay"=w462, "input_L_delayOpt"=w461, "input_T_state"=w460, "input_iSpout"=w459, "input_iTrial_relative"=w458, "input_L_T"=w439) -> ("output_LC_Event"=w457:bool, "output_LC_Laser"=w456:bool, "output_L_Tstart"=w455:u16, "output_L_Tend"=w454:u16)  [unwired: 6 in]
    }
    frame 2 {
      w469 = u16 0
      w470 = FALSE
      # "laser2 is active"
      n199 = Index Array(array=w490, index #1=w476, index #2=w475, index #3=w474, index #4=w473, index #5=w472, index #6=w471) -> (element #1=w484:u16, element #2=w485:u16, element #3=w486:u16, element #4=w487:u16, element #5=w488:u16, element #6=w489:u16)
      n200 = call "BRig_RT__Case_Exp__State_initTrial__LC.vi"("input_L_OnOff"=w484, "input_L_Block"=w485, "input_L_Count"=w486, "input_L_Prob"=w487, "input_L_Tdelay"=w488, "input_L_delayOpt"=w489, "input_T_state"=w483, "input_iSpout"=w482, "input_iTrial_relative"=w481, "input_L_T"=w468) -> ("output_LC_Event"=w478:bool, "output_LC_Laser"=w480:bool, "output_L_Tstart"=w479:u16, "output_L_Tend"=w477:u16)  [unwired: 6 in]
    }
    frame 3 {
      # "laser1 and laser2 are active"
      n201 = Index Array(array=w528, index #1=w504, index #2=w503, index #3=w502, index #4=w501, index #5=w500, index #6=w499, index #7=w498, index #8=w497, index #9=w496, index #10=w495, index #11=w494, index #12=w493) -> (element #1=w527:u16, element #2=w526:u16, element #3=w525:u16, element #4=w524:u16, element #5=w523:u16, element #6=w522:u16, element #7=w516:u16, element #8=w517:u16, element #9=w518:u16, element #10=w519:u16, element #11=w520:u16, element #12=w521:u16)
      n202 = call "BRig_RT__Case_Exp__State_initTrial__LC.vi"("input_L_OnOff"=w527, "input_L_Block"=w526, "input_L_Count"=w525, "input_L_Prob"=w524, "input_L_Tdelay"=w523, "input_L_delayOpt"=w522, "input_T_state"=w515, "input_iSpout"=w514, "input_iTrial_relative"=w513, "input_L_T"=w492) -> ("output_LC_Event"=w512:bool, "output_LC_Laser"=w511:bool, "output_L_Tstart"=w510:u16, "output_L_Tend"=w509:u16)  [unwired: 6 in]
      n203 = call "BRig_RT__Case_Exp__State_initTrial__LC.vi"("input_L_OnOff"=w516, "input_L_Block"=w517, "input_L_Count"=w518, "input_L_Prob"=w519, "input_L_Tdelay"=w520, "input_L_delayOpt"=w521, "input_T_state"=w515, "input_iSpout"=w514, "input_iTrial_relative"=w513, "input_L_T"=w491) -> ("output_LC_Event"=w506:bool, "output_LC_Laser"=w508:bool, "output_L_Tstart"=w507:u16, "output_L_Tend"=w505:u16)  [unwired: 6 in]
    }
  }
  n204 = call "BRig_dataCurrent_L_Cue_T_start_l1.vi"() -> ("outputL_Cue_T_start_l1"=w21:i32)  [unwired: 11 in]
  n205 = call "BRig_dataCurrent_L_Cue_T_end_l1.vi"() -> ("output_L_Cue_T_end_l1"=w22:i32)  [unwired: 11 in]
  n206 = call "BRig_dataCurrent_L_Cue_T_start_l2.vi"() -> ("output_L_Cue_T_start_l2"=w23:i32)  [unwired: 11 in]
  n207 = call "BRig_dataCurrent_L_Cue_T_end_l2.vi"() -> ("output_L_Cue_T_end_l2"=w24:i32)  [unwired: 11 in]
  n208 = call "BRig_dataCurrent_L_Cue2_T_start_l1.vi"() -> ("outputL_Cue2_T_start_l1"=w9:i32)  [unwired: 11 in]
  n209 = call "BRig_dataCurrent_L_Cue2_T_end_l1.vi"() -> ("output_L_Cue2_T_end_l1"=w10:i32)  [unwired: 11 in]
  n210 = call "BRig_dataCurrent_L_Cue2_T_start_l2.vi"() -> ("output_L_Cue2_T_start_l2"=w11:i32)  [unwired: 11 in]
  n211 = call "BRig_dataCurrent_L_Cue2_T_end_l2.vi"() -> ("output_L_Cue2_T_end_l2"=w12:i32)  [unwired: 11 in]
  n212 = Replace Array Subset(array="input_dataCurrent", new element #1=w107, index #1=w21, new element #2=w106, index #2=w22, new element #3=w105, index #3=w23, new element #4=w104, index #4=w24, new element #5=w82, index #5=w9, new element #6=w81, index #6=w10, new element #7=w80, index #7=w11, new element #8=w79, index #8=w12) -> (→"output_dataCurrent":u16[])
  n213 = call "BRig_dataTrial_L_Cue_event_I_l1.vi"() -> ("output_L_Cue_event_I_l1"=w1:i32)  [unwired: 11 in]
  n214 = call "BRig_dataTrial_L_Cue_trig_I_l1.vi"() -> ("output_L_Cue_trig_I_l1"=w2:i32)  [unwired: 11 in]
  n215 = call "BRig_dataTrial_L_Cue_event_I_l2.vi"() -> ("output_L_Cue_event_I_l2"=w3:i32)  [unwired: 11 in]
  n216 = call "BRig_dataTrial_L_Cue_trig_I_l2.vi"() -> ("output_L_Cue_trig_I_l2"=w4:i32)  [unwired: 11 in]
  n217 = call "BRig_dataTrial_L_Cue2_event_I_l1.vi"() -> ("output_L_Cue2_event_I_l1"=w5:i32)  [unwired: 11 in]
  n218 = call "BRig_dataTrial_L_Cue2_trig_I_l1.vi"() -> ("output_L_Cue2_trig_I_l1"=w6:i32)  [unwired: 11 in]
  n219 = call "BRig_dataTrial_L_Cue2_event_I_l2.vi"() -> ("output_L_Cue2_event_I_l2"=w7:i32)  [unwired: 11 in]
  n220 = call "BRig_dataTrial_L_Cue2_trig_I_l2.vi"() -> ("output_L_Cue2_trig_I_l2"=w8:i32)  [unwired: 11 in]
  n221 = call "BRig_arrTrig_L_Cue_event_l1.vi"() -> ("output_L_Cue_event_l1"=w13:i32)  [unwired: 11 in]
  n222 = call "BRig_arrTrig_L_Cue_laser_l1.vi"() -> ("output_L_Cue_laser_l1"=w14:i32)  [unwired: 11 in]
  n223 = call "BRig_arrTrig_L_Cue_event_l2.vi"() -> ("output_L_Cue_event_l2"=w15:i32)  [unwired: 11 in]
  n224 = call "BRig_arrTrig_L_Cue_laser_l2.vi"() -> ("output_L_Cue_laser_l2"=w16:i32)  [unwired: 11 in]
  n225 = call "BRig_arrTrig_L_Cue2_event_l1.vi"() -> ("output_L_Cue2_event_l1"=w17:i32)  [unwired: 11 in]
  n226 = call "BRig_arrTrig_L_Cue2_laser_l1.vi"() -> ("output_L_Cue2_laser_l1"=w18:i32)  [unwired: 11 in]
  n227 = call "BRig_arrTrig_L_Cue2_event_l2.vi"() -> ("output_L_Cue2_event_l2"=w19:i32)  [unwired: 11 in]
  n228 = call "BRig_arrTrig_L_Cue2_laser_l2.vi"() -> ("output_L_Cue2_laser_l2"=w20:i32)  [unwired: 11 in]
  n229 = Boolean To (0,1)(Boolean=w118) -> (0, 1=w122:i16)
  n230 = Boolean To (0,1)(Boolean=w115) -> (0, 1=w121:i16)
  n231 = Boolean To (0,1)(Boolean=w113) -> (0, 1=w119:i16)
  n232 = Boolean To (0,1)(Boolean=w111) -> (0, 1=w120:i16)
  n233 = Boolean To (0,1)(Boolean=w86) -> (0, 1=w98:i16)
  n234 = Boolean To (0,1)(Boolean=w85) -> (0, 1=w97:i16)
  n235 = Boolean To (0,1)(Boolean=w84) -> (0, 1=w95:i16)
  n236 = Boolean To (0,1)(Boolean=w83) -> (0, 1=w96:i16)
  n237 = Replace Array Subset(array="input_arrTrig", new element #1=w118, index #1=w13, new element #2=w115, index #2=w14, new element #3=w113, index #3=w15, new element #4=w111, index #4=w16, new element #5=w86, index #5=w17, new element #6=w85, index #6=w18, new element #7=w84, index #7=w19, new element #8=w83, index #8=w20) -> (→"output_arrTrig":bool[])
  n238 = To Unsigned Word Integer(number=w122) -> (unsigned 16bit integer=w117:u16)
  n239 = To Unsigned Word Integer(number=w121) -> (unsigned 16bit integer=w116:u16)
  n240 = To Unsigned Word Integer(number=w119) -> (unsigned 16bit integer=w114:u16)
  n241 = To Unsigned Word Integer(number=w120) -> (unsigned 16bit integer=w112:u16)
  n242 = To Unsigned Word Integer(number=w98) -> (unsigned 16bit integer=w93:u16)
  n243 = To Unsigned Word Integer(number=w97) -> (unsigned 16bit integer=w92:u16)
  n244 = To Unsigned Word Integer(number=w95) -> (unsigned 16bit integer=w91:u16)
  n245 = To Unsigned Word Integer(number=w96) -> (unsigned 16bit integer=w90:u16)
  n246 = Replace Array Subset(array="input_dataTrial", new element #1=w117, index (row) #1=w94, index (col) #1=w1, new element #2=w116, index (row) #2=w94, index (col) #2=w2, new element #3=w114, index (row) #3=w94, index (col) #3=w3, new element #4=w112, index (row) #4=w94, index (col) #4=w4, new element #5=w93, index (row) #5=w94, index (col) #5=w5, new element #6=w92, index (row) #6=w94, index (col) #6=w6, new element #7=w91, index (row) #7=w94, index (col) #7=w7, new element #8=w90, index (row) #8=w94, index (col) #8=w8) -> (→"output_dataTrial":u16[][])
